vi "Get Static Channel Reference for Frame.vi"(8 "error in":errorcluster, 11 "label ref":T1 format="%.0x") -> (0 "error out":errorcluster, 2 "channel specification ref":T1 format="%.0x", 3 "label ref out":T1 format="%.0x", 4 "found?":bool)   [LabVIEW 2020]
uses:
  <vilib>/NI VeriStand/Custom Device API/Custom Device Item Ref.ctl
  Scripting/Constants.vi
  <vilib>/NI VeriStand/Custom Device Tools/Custom Device Utility Library/NI VeriStand - Search for Item by GUID.vi
  <vilib>/NI VeriStand/Custom Device Tools/Custom Device Utility Library/Custom Device Utility Library.lvlib
  Scripting/Ballard ARINC 429 Scripting.lvlib
  <vilib>/NI VeriStand/Custom Device API/Custom Device API.lvlib
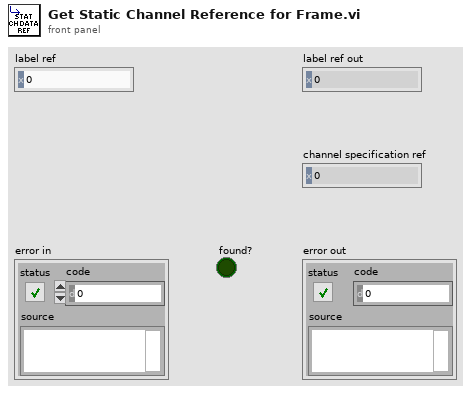
[diagram p1: front panel]
types:
  T1 = typedef "Custom Device API.lvlib/Custom Device Item Ref.ctl" = u64
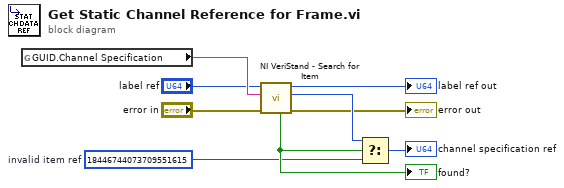
[diagram p0: block diagram]
diagram:
  w1 = T1 18446744073709551615  # invalid item ref
  n1 = global read "Constants.vi" "GUID.Channel Specification"() -> (w9:string)
  n2 = call-poly <vilib>:"NI VeriStand - Search for Item.vi"("error in"="error in", "Item GUID"=w9, "Section Ref in"="label ref") -> ("error out"=→"error out":errorcluster, "Item Ref"=w7:T1, "Section Ref out"=→"label ref out":T1, "Found"=w6:bool)  [unwired: 5 in]
  "found?" <- w6
  n3 = Select(t=w7, s=w6, f=w1) -> (s? t:f=→"channel specification ref":T1)
